vi "Set Bucket Versioning.vi"(7 "Auth device data":T1, 8 "error in (no error)":errorcluster, 9 "MFA Delete":T2, 10 "Status":T3, 11 "Bucket in":refnum<class "Bucket.lvclass">) -> (0 "error out":errorcluster, 3 "Bucket out":refnum<class "Bucket.lvclass">)   [LabVIEW 2015, in "NI_AWS_S3.lvlib" / "Bucket.lvclass"]
uses:
  Bucket.lvclass
  Versioning Status.ctl
  MFA Delete.ctl
  Auth Device Data.ctl
  Core/HTTP Request/Region handling.ctl
  Core/HTTP Request/Request Options.ctl
  Core/HTTP Request/Name Value Pair.ctl
  Core/HTTP Request/URL formatting.ctl
  Bucket.lvclass/Bucket.ctl
  Read Name.vi
  Core/HTTP Request/HTTP Request.lvclass
  NI_AWS_S3.lvlib
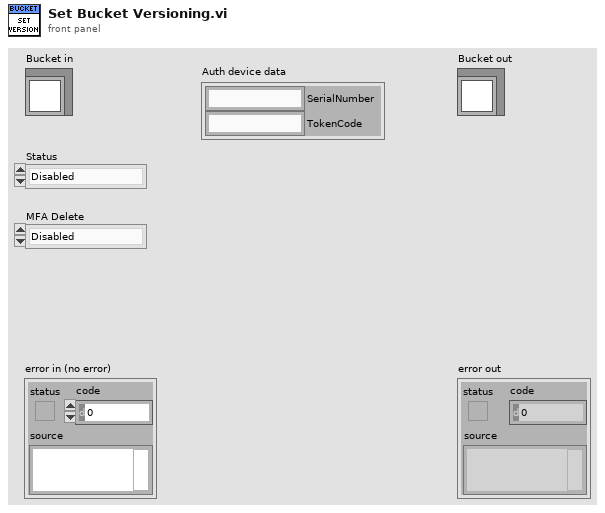
[diagram p1: front panel]
types:
  T1 = typedef "NI_AWS_S3.lvlib/Auth Device Data.ctl" = cluster{"SerialNumber":string, "TokenCode":string}
  T2 = typedef "NI_AWS_S3.lvlib/Bucket.lvclass/MFA Delete.ctl" = enum16{"Disabled", "Enabled"}
  T3 = typedef "NI_AWS_S3.lvlib/Bucket.lvclass/Versioning Status.ctl" = enum16{"Disabled", "Suspended", "Enabled"}
  T4 = typedef "NI_AWS_Core.lvlib/HTTP Request.lvclass/Name Value Pair.ctl" = cluster{"name":string, "value":string}
  T5 = typedef "NI_AWS_Core.lvlib/HTTP Request.lvclass/Request Options.ctl" = cluster{"request headers":T4[], "request parameters":T4[], "request body":string, "region handling":T6, "URL formatting":T7}
  T6 = typedef "NI_AWS_Core.lvlib/HTTP Request.lvclass/Region handling.ctl" = enum16{"use region everywhere", "use region (authentication only)", "use region (URL only)", "ignore region everwhere"}
  T7 = typedef "NI_AWS_Core.lvlib/HTTP Request.lvclass/URL formatting.ctl" = enum16{"region-", "region."}
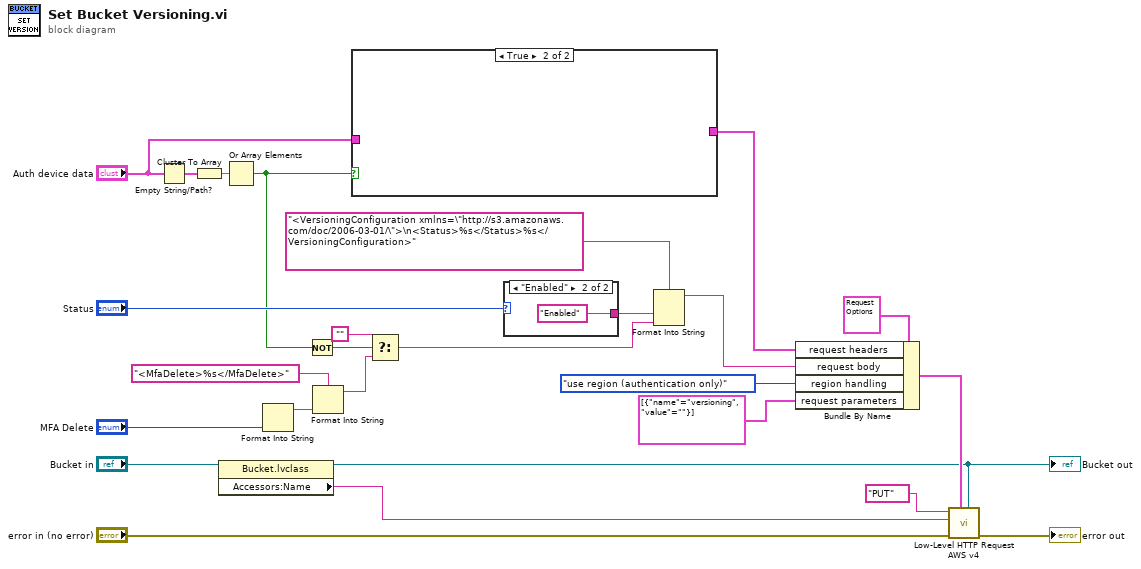
[diagram p0: block diagram]
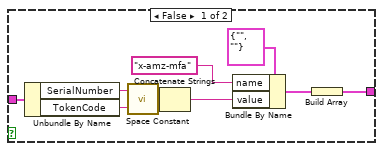
[diagram p2: hidden frame]
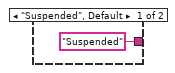
[diagram p3: hidden frame]
diagram:
  n1 = Empty String/Path?(string/path="Auth device data") -> (empty?=w6:cluster{"SerialNumber":bool, "TokenCode":bool})
  n2 = Cluster To Array(cluster=w6) -> (array=w7:bool[])
  n3 = property class="Bucket.lvclass"(reference="Bucket in") -> (reference out=w20:refnum<class "Bucket.lvclass">, "Accessors:Name"=w25:string)  [unwired: 1 in, 1 out]
  "Bucket out" <- w20
  n4 = Or Array Elements(Boolean array=w7) -> (logical OR=w4:bool)
  n5 = Format Into String("MFA Delete") -> (resulting string=w9:string)  [unwired: 3 in, 1 out]
  n6 = Not(x=w4) -> (.not. x?=w1:bool)
  n7 = Format Into String(format string="<MfaDelete>%s</MfaDelete>", w9) -> (resulting string=w8:string)  [unwired: 2 in, 1 out]
  n8 = case shown="True" w4 {
    tunnel: "Auth device data" -> [w30 _]
    tunnel: [w28 _] -> w2
    frame False {
      n9 = Unbundle By Name(w30) -> ("SerialNumber"=w35:string, "TokenCode"=w34:string)
      n10 = call <vilib>:"Space Constant.vi"() -> ("String"=w33:string)
      n11 = Concatenate Strings(w35, w33, w34) -> (w32:string)
      n12 = Bundle By Name(cluster=T4 {"name"="", "value"=""} ("Name Value Pair"), "name"="x-amz-mfa" ("Header"), "value"=w32) -> (w29:T4)
      n13 = Build Array(w29) -> (w28:T4[])
    }
    frame True {
    }
  }
  n14 = Select(t="", s=w1, f=w8) -> (s? t:f=w11:string)
  n15 = case shown="\"Enabled\"" "Status" {
    tunnel: ["Suspended" "Enabled"] -> w12
    frame "Suspended", Default {
    }
    frame "Enabled" {
    }
  }
  n16 = Format Into String(format string="<VersioningConfiguration xmlns=\"http://s3.amazonaws.com/doc/2006-03-01/\">\n<Status>%s</Status>%s</VersioningConfiguration>", w12, w11) -> (resulting string=w3:string)  [unwired: 2 in, 1 out]
  n17 = Bundle By Name(cluster=T5 {"request headers"=[], "request parameters"=[], "request body"="", "region handling"=enum."use region everywhere", "URL formatting"=enum."region."} ("Request Options"), "request headers"=w2, "request body"=w3, "region handling"=Region_handling."use region (authentication only)", "request parameters"=T4[] [{"name"="versioning", "value"=""}]) -> (w22:T5)
  n18 = call "Low-Level HTTP Request AWS v4.vi"("AWS Core"=w20, "Request Options"=w22, "error in (no error)"="error in (no error)", "URL Prefix"=w25, "HTTP-Verb"="PUT") -> ("error out"=→"error out":errorcluster)  [unwired: 4 in, 2 out]
